vi "Send Mixed Mode Command.vi"(0 "Targets":T1[](array[typedef]), 1 "MCL Command In":refnum<queue>, 2 "Ramp Times":cluster{"Displacement":T3, "Force":T3}, 3 "error in":errorcluster) -> (5 "MCL Command Out":refnum<queue>, 6 "error out":errorcluster)   [LabVIEW 2009]
uses:
  Ramp Time Tuple.ctl
  Messages/Mixed Mode Command.ctl
  Mixed Mode Command Action.ctl
  Target Data.ctl
  Data Access Objects/Metadata/LBCB Space.ctl
  Target.ctl
  Data Access Objects/Metadata/LBCB Number.ctl
  Apps/App Status Actions.ctl
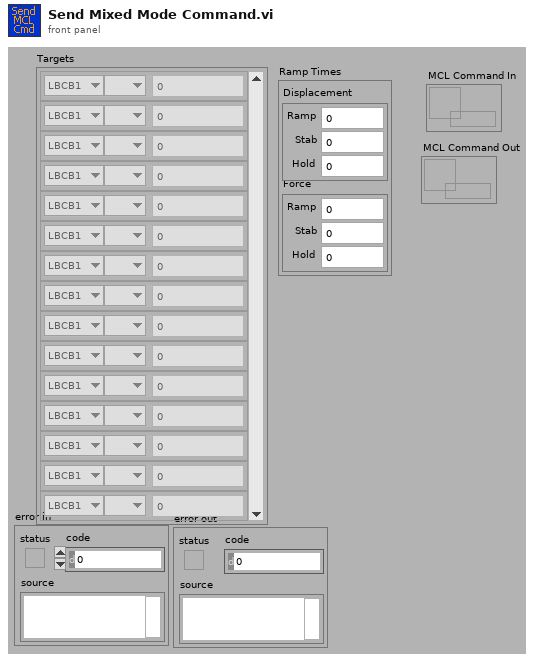
[diagram p1: front panel]
types:
  T1 = typedef "Target.ctl" = cluster{"LBCB Number":T2, "DOF Vectors":enum16{" ", "Dx", "Dy", "Dz", "Rx", "Ry", "Rz", "Fx", "Fy", "Fz", "Mx", "My", "Mz"}, "Amount":dbl}
  T2 = typedef "LBCB Number.ctl" = enum16{"LBCB1", "LBCB2"}
  T3 = typedef "Ramp Time Tuple.ctl" = cluster{"Ramp":dbl, "Stab":dbl, "Hold":dbl}
  T4 = typedef "Mixed Mode Command.ctl" = cluster{"Command":T5, "Ramp Times":cluster{"Initial":T3, "Iterative":T3}, "LBCB1":T6, "LBCB2":T6}
  T5 = typedef "Mixed Mode Command Action.ctl" = enum16{"Start Command", "Stop", "Exit", "No Op", "Start Acquisition", "Measure Initial Position"}
  T6 = typedef "Target Data.ctl" = cluster{"Displacements":dbl[], "Command Type":enum16{"<None>", "Displacement", "Force"}[], "Forces":dbl[], "Space":T7}
  T7 = typedef "LBCB Space.ctl" = enum16{"Actuator", "Cartesian"}
  T8 = typedef "App Status Actions.ctl" = enum16{"Init", "Get Status", "Running", "Control", "Autobalanced", "Data Acquisition", "Set App State", "DAQ Started", "Set LBCB State", "Set All", "Set Cont Logging", "Set Step Logging", "Set MM Logging", "Set Volt Logging", "Set Cart Type", "Set DAQ Link", "Set NTCP Link"}
  T9 = typedef "App Status.ctl" = cluster{"Running":bool, "Controlling L2":bool, "Autobalance L2":bool, "Data Acquisition":bool, " App State":T10, "DAQ Started":bool, "LBCB 1 State":T11, "LBCB 2 State":T11, "Controlling L1":bool, "Autobalance L1":bool, "Cartesian Type":bool, "Continuous Logging":bool, "Step Logging":bool, "Voltage Logging":bool, "Mixed Mode Logging":bool, "DAQ Link":bool, "NTCP Link ":bool}
  T10 = typedef "AppStates.ctl" = enum16{"Starting OM", "Initializing Displays", "Setting up Archiving", "Setting Up DAQ Channels", "Start DAQ", "DAQ Starting", "Controlling LBCBs", "Stopping OM"}
  T11 = typedef "Lbcb Control Loop States.ctl" = enum16{"Idle", "Start Selected", "Load Last Command", "Start Autobalancing", "Autobalancing", "Control Loop Initialized", "Control Enabled"}
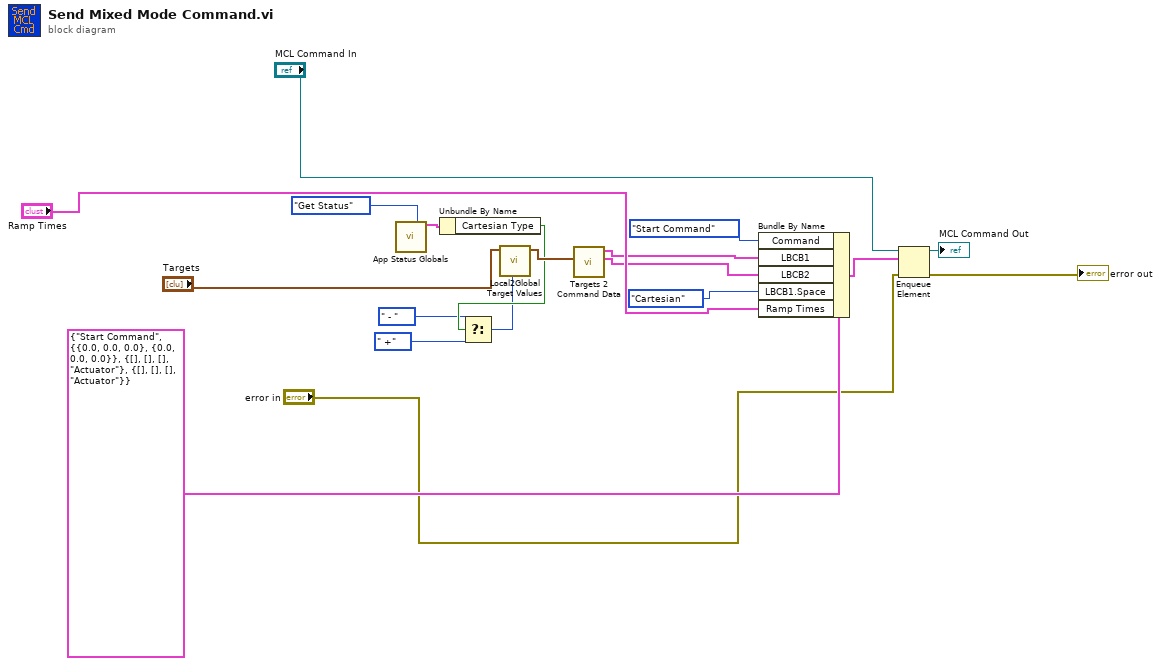
[diagram p0: block diagram]
diagram:
  n1 = call "App Status Globals.vi"("App Status Actions"=App_Status_Actions."Get Status") -> ("App Status Out"=w4:T9)  [unwired: 5 in, 9 out]
  n2 = Unbundle By Name(w4) -> ("Cartesian Type"=w8:bool)
  n3 = Select(t=enum16{" +", " - "}." - " ("Direction"), s=w8, f=enum16{" +", " - "}." +") -> (s? t:f=w6:enum16{" +", " - "})
  n4 = call "Local2Global Target Values.vi"("Direction"=w6, "Target  Inputs"="Targets") -> ("Target  Outputs"=w9:T1[])  [unwired: 9 in]
  n5 = call "Targets 2 Command Data.vi"("Target  Inputs"=w9) -> ("LBCB 2 Command Data"=w13:T6, "LBCB 1 Command Data"=w12:T6)  [unwired: 9 out]
  n6 = Bundle By Name(cluster=T4 {"Command"=enum."Start Command", "Ramp Times"={"Initial"={"Ramp"=0.0, "Stab"=0.0, "Hold"=0.0}, "Iterative"={"Ramp"=0.0, "Stab"=0.0, "Hold"=0.0}}, "LBCB1"={"Displacements"=[], "Command Type"=[], "Forces"=[], "Space"=enum."Actuator"}, "LBCB2"={"Displacements"=[], "Command Type"=[], "Forces"=[], "Space"=enum."Actuator"}} ("Mixed Mode Command In"), "Command"=Mixed_Mode_Command_Action."Start Command", "LBCB1"=w12, "LBCB2"=w13, "LBCB1.Space"=LBCB_Space."Cartesian" ("Space"), "Ramp Times"="Ramp Times") -> (w14:T4)
  n7 = Enqueue Element(queue="MCL Command In", element=w14, error in (no error)="error in") -> (queue out=→"MCL Command Out":refnum<queue>, error out=→"error out":errorcluster)  [unwired: 1 in, 1 out]
